vi "ControlMotorCalculatePusle.vi"(3 "数据":dbl, 4 "计算状态":enum32{"位置-脉冲", "脉冲-位置"}(radio), 5 "控制电机":T2) -> (1 "dataout":dbl)   [LabVIEW 2018]
panel:
  in  "簇":T1
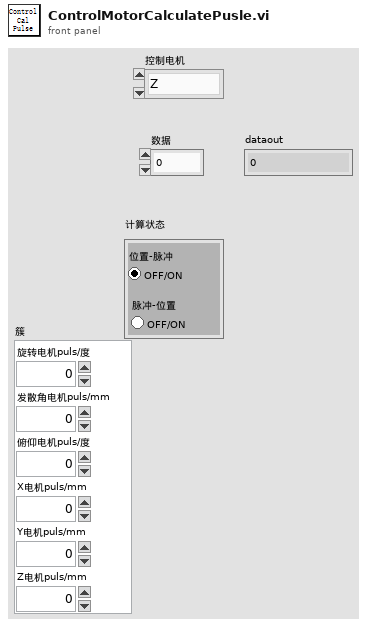
[diagram p1: front panel]
types:
  T1 = cluster{"旋转电机puls/度":dbl, "发散角电机puls/mm":i32, "俯仰电机puls/度":dbl, "X电机puls/mm":i32, "Y电机puls/mm":i32, "Z电机puls/mm":i32}
  T2 = typedef "控制电机枚举器.ctl" = enum16{"Z", "Y", "X", "发散角", "俯仰", "旋转"}
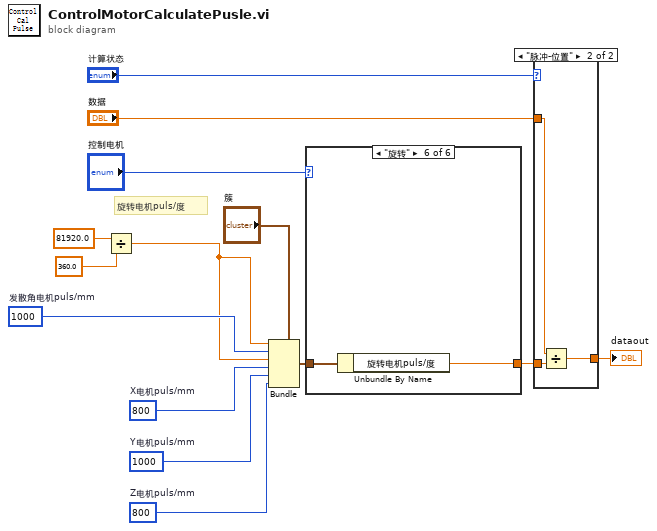
[diagram p0: block diagram]
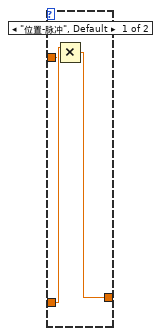
[diagram p2: hidden frame]
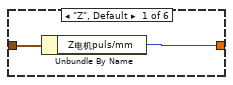
[diagram p3: hidden frame]
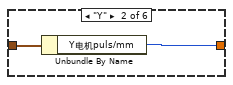
[diagram p4: hidden frame]
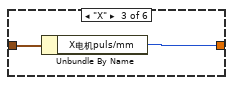
[diagram p5: hidden frame]
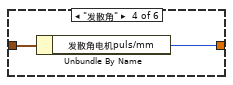
[diagram p6: hidden frame]
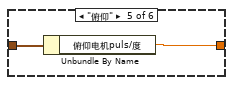
[diagram p7: hidden frame]
diagram:
  w11 = 800  # Z电机puls/mm
  w12 = 1000  # Y电机puls/mm
  w13 = 800  # X电机puls/mm
  w14 = 1000  # 发散角电机puls/mm
  # "旋转电机puls/度"
  n1 = Divide(x=81920.0, y=360.0) -> (x/y=w1:dbl)
  n2 = Bundle(cluster="簇", "旋转电机puls/度"=w1, "发散角电机puls/mm"=w14, "俯仰电机puls/度"=w1, "X电机puls/mm"=w13, "Y电机puls/mm"=w12, "Z电机puls/mm"=w11) -> (w10:T1)
  n3 = case shown="\"旋转\"" "控制电机" {
    tunnel: w10 -> [w16 w18 w20 w22 w24 w26]
    tunnel: [w15 w17 w19 w21 w23 w25] -> w8
    frame "Z", Default {
      n4 = Unbundle By Name(w16) -> ("Z电机puls/mm"=w15:i32)
    }
    frame "Y" {
      n5 = Unbundle By Name(w18) -> ("Y电机puls/mm"=w17:i32)
    }
    frame "X" {
      n6 = Unbundle By Name(w20) -> ("X电机puls/mm"=w19:i32)
    }
    frame "发散角" {
      n7 = Unbundle By Name(w22) -> ("发散角电机puls/mm"=w21:i32)
    }
    frame "俯仰" {
      n8 = Unbundle By Name(w24) -> ("俯仰电机puls/度"=w23:dbl)
    }
    frame "旋转" {
      n9 = Unbundle By Name(w26) -> ("旋转电机puls/度"=w25:dbl)
    }
  }
  n10 = case shown="\"脉冲-位置\"" "计算状态" {
    tunnel: w8 -> [w29 w30]
    tunnel: [w27 w32] -> w7
    tunnel: "数据" -> [w28 w31]
    frame "位置-脉冲", Default {
      n11 = Multiply(x=w29, y=w28) -> (x*y=w27:dbl)
    }
    frame "脉冲-位置" {
      n12 = Divide(x=w31, y=w30) -> (x/y=w32:dbl)
    }
  }
  "dataout" <- w7
